vi "GenerateSTP_FlowControlPayload.vi"(8 "error in (no error)":errorcluster, 10 "SeperationTime(ST)":u8, 11 "BlockSize(BS)":u8) -> (0 "error out":errorcluster, 3 "Flow Control Payload":u8[](array[numeric]))   [LabVIEW 2023, in "HardwareAbstractionLayer_LVOOP.lvlib" / "CAN Application Protocols Lib.lvlib" / "STP Protocol.lvclass"]
uses:
  STP Protocol.lvclass
  Ctrls/TP Frame Type.ctl
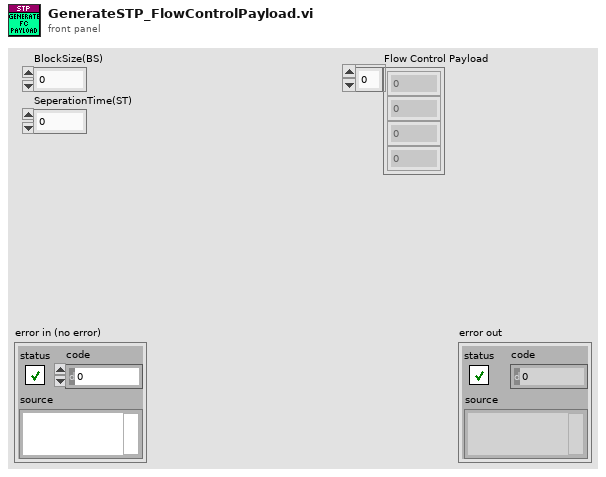
[diagram p1: front panel]
types:
  T1 = typedef "HardwareAbstractionLayer_LVOOP.lvlib/CAN Application Protocols Lib.lvlib/STP Protocol.lvclass/TP Frame Type.ctl" = u8
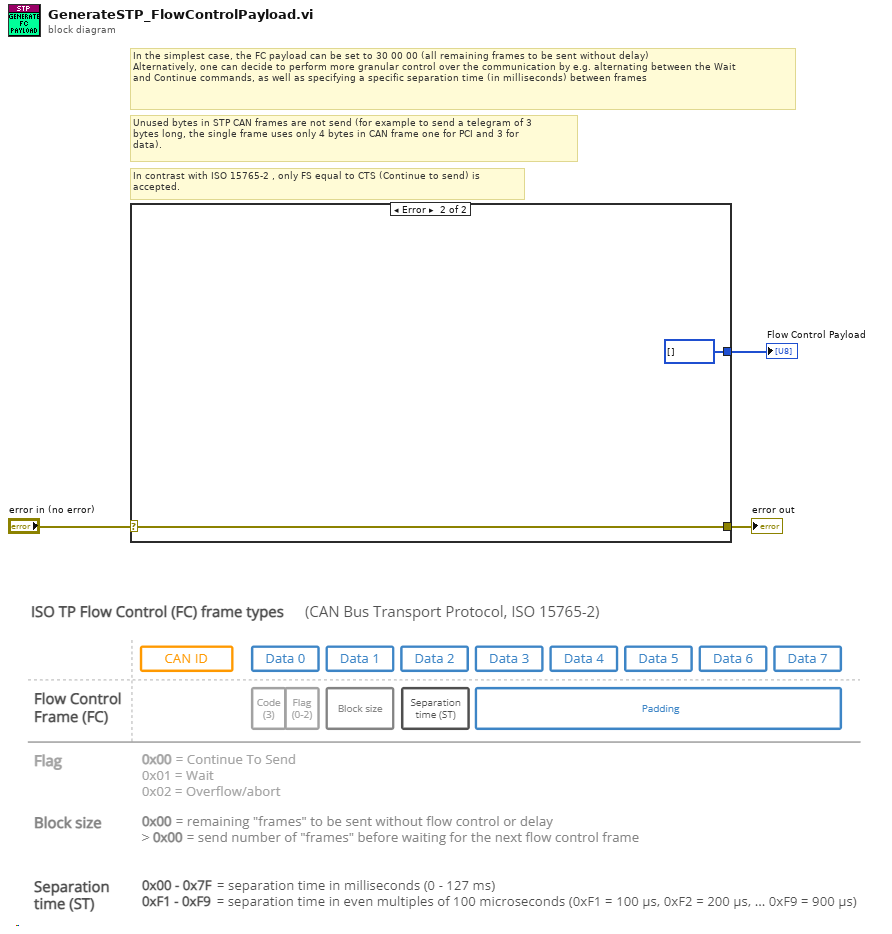
[diagram p0: block diagram]
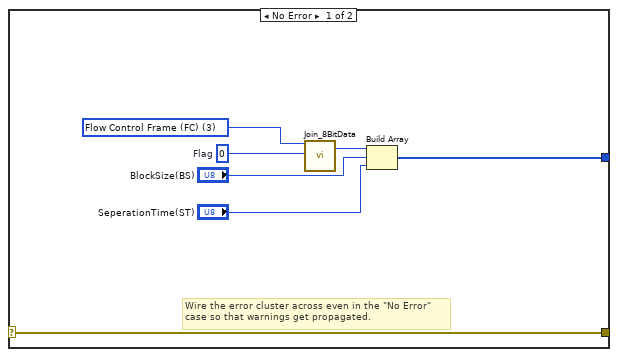
[diagram p2: hidden frame]
diagram:
  # "In contrast with ISO 15765-2 , only FS equal to CTS (Continue to send) is\naccepted."
  # "Unused bytes in STP CAN frames are not send (for example to send a telegram of 3\nbytes long, the single frame uses only 4 bytes in CAN frame one for PCI and 3 for\ndata)."
  # "In the simplest case, the FC payload can be set to 30 00 00 (all remaining frames to be sent without delay)\nAlternatively, one can decide to perform more granular control over the communication by e.g. alternating between the Wait \nand Continue commands, as well as specifying a specific separation time (in milliseconds) between frames"
  n1 = case shown="Error" "error in (no error)" {
    selector: "error in (no error)" -> [w10 w12]
    tunnel: [w10 w12] -> w2
    tunnel: [w4 u8[] []] -> w1
    frame No Error {
      w8 = u8 0  # Flag
      w9 = T1 3 items=["Single Frame (SF)", "First Frame (SF)", "Consecutive Frame (CF)", "Flow Control Frame (FC)"] ("Ring")
      # "Wire the error cluster across even in the \"No Error\"\ncase so that warnings get propagated."
      n2 = call "Join_8BitData.vi"("hi"=w9, "lo"=w8) -> ("hi.lo(8bits)"=w7:u8)  [unwired: 17 in]
      n3 = Build Array(w7, "BlockSize(BS)", "SeperationTime(ST)") -> (w4:u8[])
    }
    frame Error {
    }
  }
  "error out" <- w2
  "Flow Control Payload" <- w1
